vi "CS++Test.vi"() -> ()   [LabVIEW 2013]
uses:
  CSPP_Core/Classes/CS++BaseClasses/Factory/CS++Factory.lvclass
  CSPP_Core/Classes/CS++ProcessVariables/PVConnection/PVConnection.lvclass
  CSPP_Core/Classes/CS++ProcessVariables/ProcessVariable/PV.lvclass
  CSPP_Core/Classes/CS++ProcessVariables/ProcessVariable/PV.lvclass/PV.ctl
  CSPP_Core/Classes/CS++BaseClasses/Factory/CS++Factory.lvclass/CS++Factory.ctl
  CSPP_Core/Classes/CS++ProcessVariables/ProcessVariable/Write Data.vi
  CSPP_Core/Classes/CS++ProcessVariables/ProcessVariable/Read Data.vi
  CSPP_Core/Classes/CS++ProcessVariables/ProcessVariable/Read Error.vi
  CSPP_Core/Classes/CS++ProcessVariables/ProcessVariable/Read PV URL.vi
  CSPP_Core/Classes/CS++ProcessVariables/ProcessVariable/Read Quality.vi
  CSPP_Core/Classes/CS++ProcessVariables/ProcessVariable/Read status.vi
  CSPP_Core/Classes/CS++ProcessVariables/ProcessVariable/Read Timestamp.vi
panel:
  out "timestamp":timestamp
  out "status":u32
  out "quality":u64
  out "PV URL":string
  out "Error In":errorcluster
  out "data":variant
  in  "File Path Control":path=path "C:/User/Brand/LVP/CSPP/Packages/CSPP_Examples/CS++Example.ini"
  in  "Object Name":string="mySV"
  out "Attributes found?":bool
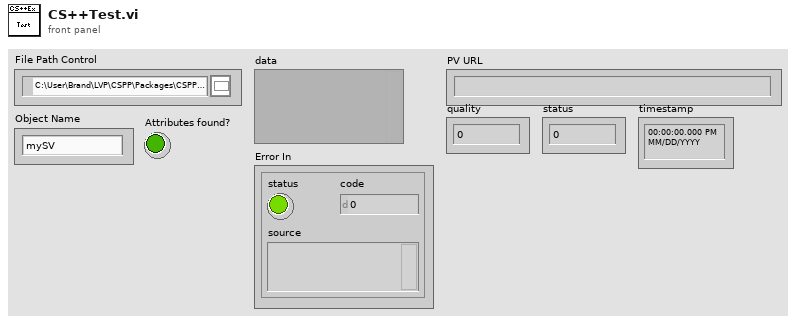
[diagram p1: front panel]
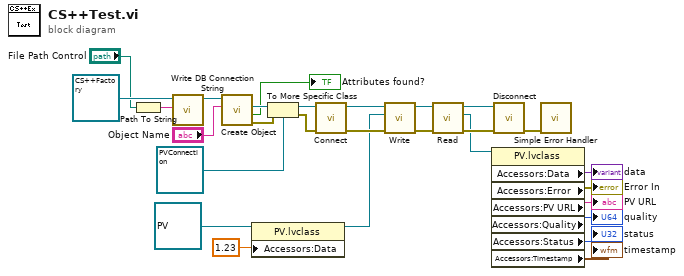
[diagram p0: block diagram]
diagram:
  n1 = Path To String(path="File Path Control") -> (string=w9:string)
  n2 = call "Write DB Connection String.vi"("DB Connection String"=w9, "CS++Factory in"=refnum<class "CS++Factory.lvclass"> refnum ("CS++BaseClasses.lvlib:CS++Factory.lvclass")) -> ("CS++Factory out"=w10:refnum<class "CS++Factory.lvclass">)  [unwired: 8 in, 1 out]
  n3 = call "Create Object.vi"("Object Name"="Object Name", "CS++Factory in"=w10) -> ("error out"=w27:errorcluster, "Attributes found?"=→"Attributes found?":bool, "LabVIEW Object"=w28:refnum<class>)  [unwired: 6 in, 1 out]
  n4 = property class="PV.lvclass"(reference=refnum<class "PV.lvclass"> refnum ("CS++ProcessVariables.lvlib:PV.lvclass"), "Accessors:Data"=1.23) -> (reference out=w17:refnum<class "PV.lvclass">)  [unwired: 1 in, 1 out]
  n5 = To More Specific Class(target class=refnum<class "PVConnection.lvclass"> refnum ("CS++ProcessVariables.lvlib:PVConnection.lvclass"), reference=w28, error in=w27) -> (specific class reference=w23:refnum<class "PVConnection.lvclass">, error out=w22:errorcluster)
  n6 = call-dynamic "Connect.vi"("error in (no error)"=w22, "PVConnection in"=w23) -> ("error out"=w20:errorcluster, "PVConnection out"=w21:refnum<class "PVConnection.lvclass">)  [unwired: 8 in]
  n7 = call-dynamic "Write.vi"("error in (no error)"=w20, "PV"=w17, "PVConnection in"=w21) -> ("error out"=w15:errorcluster, "PVConnection out"=w16:refnum<class "PVConnection.lvclass">)  [unwired: 7 in]
  n8 = call-dynamic "Read.vi"("error in (no error)"=w15, "PVConnection in"=w16) -> ("error out"=w13:errorcluster, "PV"=w7:refnum<class "PV.lvclass">, "PVConnection out"=w14:refnum<class "PVConnection.lvclass">)  [unwired: 7 in]
  n9 = property class="PV.lvclass"(reference=w7) -> ("Accessors:Data"=→"data":variant, "Accessors:Error"=→"Error In":errorcluster, "Accessors:PV URL"=→"PV URL":string, "Accessors:Quality"=→"quality":i32, "Accessors:Status"=→"status":i32, "Accessors:Timestamp"=→"timestamp":timestamp)  [unwired: 1 in, 2 out]
  n10 = call-dynamic "Disconnect.vi"("error in (no error)"=w13, "PVConnection in"=w14) -> ("error out"=w12:errorcluster)  [unwired: 8 in, 1 out]
  n11 = call <vilib>:"Simple Error Handler.vi"("error in (no error)"=w12) -> ()  [unwired: 4 in, 5 out]
